vi "API ID.vi"(11 "TelemetryAPI in":refnum<class "TelemetryAPI.lvclass">) -> (2 "ID":string)   [LabVIEW 2020, in "Volatus.lvlib" / "TelemetryAPI.lvclass"]
uses:
  TelemetryAPI.lvclass
  TelemetryAPI.lvclass/TelemetryAPI.ctl
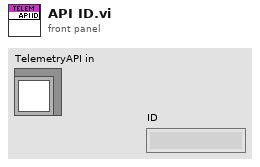
[diagram p1: front panel]
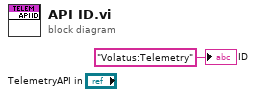
[diagram p0: block diagram]
diagram:
  "ID" <- "Volatus:Telemetry" ("ID")
